vi "replace_in_stringSD.vi"(2 "error in (no error)":errorcluster, 3 "replaced to..":string=";", 4 "characters to replace":string="[ \\t]+", 5 "input string":string="   \t\ttry    this 22  32  \t\t\n  newline\n 32 38   322323 \nfshvc    \t") -> (0 "error out":errorcluster, 1 "output string":string)   [LabVIEW 2020]
panel:
  # "[ \\t]+ matches space and tab but not newline"
  # "[\\s]+ matches space, tab, newline, carriage return, and so on"
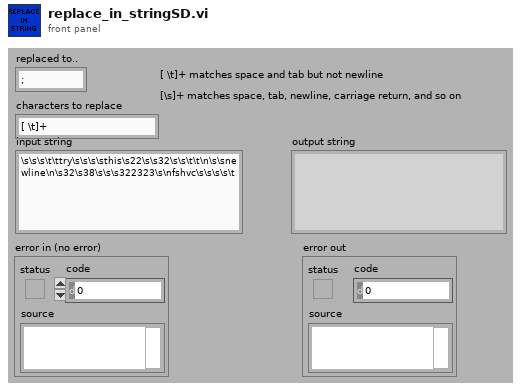
[diagram p1: front panel]
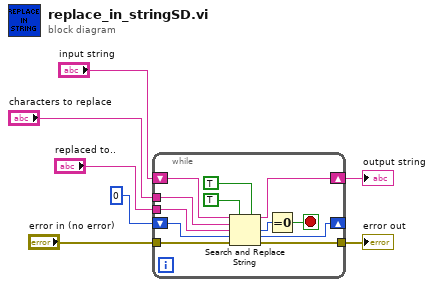
[diagram p0: block diagram]
diagram:
  n1 = while {
    tunnel: "characters to replace" -> [w19]
    tunnel: "replaced to.." -> [w18]
    shift-right: [w16] -> _
    shift-left: 0 -> [w17]
    shift-right: [w12] -> w3
    shift-left: "input string" -> [w13]
    tunnel: "error in (no error)" -> [w9]
    tunnel: [w8] -> w1
    stop <- w14 stop-if-true
    n2 = Search and Replace String(replace all?=TRUE ("replace all? (F)"), multiline?=TRUE ("multiline? (F)"), input string=w13, search string=w19, replace string=w18, offset=w17, error in=w9) -> (result string=w12:string, number of replacements=w15:i32, offset past replacement=w16:i32, error out=w8:errorcluster)  [unwired: 1 in]
    n3 = Equal To 0?(x=w15) -> (x = 0?=w14:bool)
  }
  "output string" <- w3
  "error out" <- w1
